vi "XYdata remove zero reduce pts.vi"(5 "reduce data pts":bool, 6 "# of final data pts":i32=5000, 7 "replace with interp. data":bool, 8 "iteration number":i32, 9 "remove zero":bool, 11 "2D input":dbl[][](array[numeric])) -> (3 "2D output":dbl[][](array[numeric]))   [LabVIEW 2020]
panel:
  # "Filter 1: Speed mode ON or OFF\nFileter 2: Remove Zero On or OFF\n    Replace with interp. data ON/OFF: When filter 2 is ON, the removed data were replaced by interpolated data"
  # "Caution: All rows will be affected."
  # "(1) Select datasets to be processed"
  # "(2) Reduce # of data if desired"
  # "(3) Select parameters for removing zeros"
  # "i) run zero-removing process?"
  # "ii) chose target column or perform for all columns"
  # "ii) after processing"
  # "delete data pts"
  # "(3) Start processing"
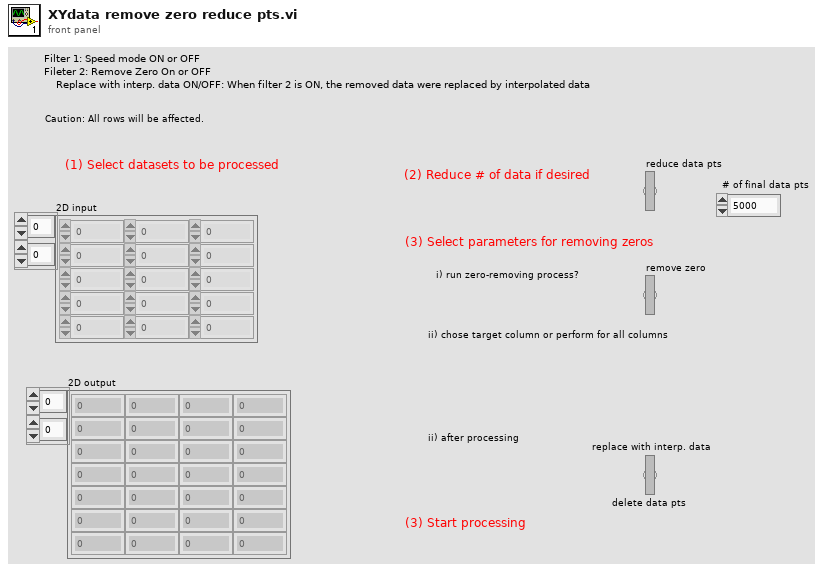
[diagram p1: front panel]
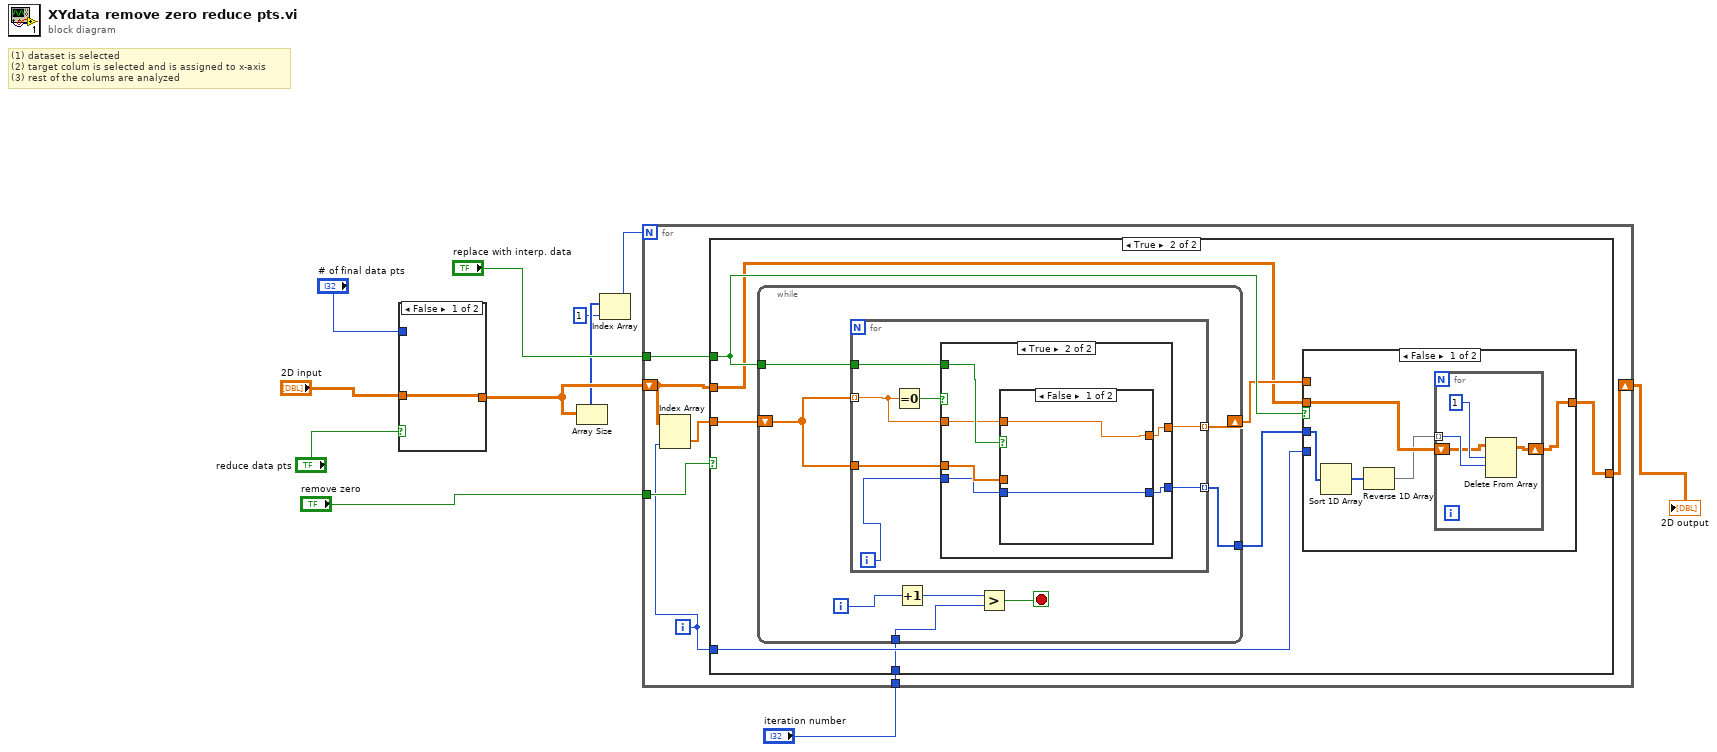
[diagram p0: block diagram]
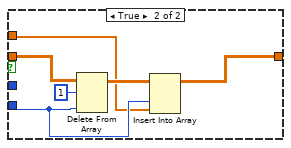
[diagram p3: hidden frame]
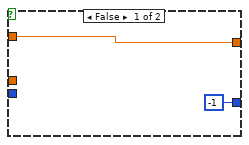
[diagram p4: hidden frame]
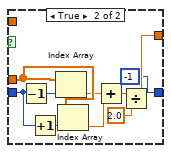
[diagram p5: hidden frame]
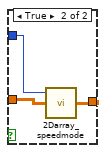
[diagram p6: hidden frame]
diagram:
  # "(1) dataset is selected\n(2) target colum is selected and is assigned to x-axis\n(3) rest of the colums are analyzed"
  n1 = case shown="False" "reduce data pts" {
    tunnel: [w12 w15] -> w8
    tunnel: "# of final data pts" -> [_ w14]
    tunnel: "2D input" -> [w12 w13]
    frame False {
    }
    frame True {
      n2 = call "2Darray_speedmode.vi"("original 2D array"=w13, "# of rows"=w14) -> ("reduced 2D array"=w15:dbl[][])  [unwired: 1 in]
    }
  }
  n3 = Array Size(array=w8) -> (size(s)=w3:i32[])
  n4 = Index Array(array=w3, index=1) -> (element=w1:i32)
  n5 = for {
    N: w1 -> [_]
    tunnel: "remove zero" -> [w22]
    tunnel: "replace with interp. data" -> [w21]
    tunnel: "iteration number" -> [w20]
    shift-right: [w19] -> w4
    shift-left: w8 -> [w16]
    i -> [w17]
    n6 = Index Array(array=w16, index (col)=w17) -> (element=w18:dbl[])  [unwired: 1 in]
    n7 = case shown="True" w22 {
      tunnel: w18 -> [_ w31]
      tunnel: [w23 w28] -> w19
      tunnel: w21 -> [_ w30]
      tunnel: w16 -> [w23 w26]
      tunnel: w17 -> [_ w25]
      tunnel: w20 -> [_ w24]
      frame False {
      }
      frame True {
        n8 = while {
          shift-right: [w53] -> w29
          shift-left: w31 -> [w54]
          tunnel: w30 -> [w49]
          tunnel: [w48] -> w27
          tunnel: w24 -> [w47]
          i -> [w52]
          stop <- w51 stop-if-true
          n9 = for {
            tunnel: w54 -> [w60] mode=indexing
            tunnel: [w61] -> w53 mode=indexing
            tunnel: w54 -> [w59]
            tunnel: w49 -> [w57]
            tunnel: [w56] -> w48 mode=indexing
            i -> [w58]
            n10 = Equal To 0?(x=w60) -> (x = 0?=w55:bool)
            n11 = case shown="True" w55 {
              tunnel: [w63 w64] -> w61
              tunnel: w60 -> [w63 w65]
              tunnel: w59 -> [_ w69]
              tunnel: w58 -> [_ w68]
              tunnel: w57 -> [_ w67]
              tunnel: [-1 w66] -> w56
              frame False {
              }
              frame True {
                n12 = case shown="False" w67 {
                  tunnel: w69 -> [_ w81]
                  tunnel: w68 -> [w71 w80]
                  tunnel: [w70 w73] -> w64
                  tunnel: [w71 -1] -> w66
                  tunnel: w65 -> [w70 _]
                  frame False {
                  }
                  frame True {
                    n13 = Decrement(x=w80) -> (x-1=w79:i32)
                    n14 = Increment(x=w80) -> (x+1=w78:i32)
                    n15 = Index Array(array=w81, index=w79) -> (element=w77:dbl)
                    n16 = Index Array(array=w81, index=w78) -> (element=w76:dbl)
                    n17 = Add(x=w77, y=w76) -> (x+y=w75:dbl)
                    n18 = Divide(x=w75, y=2.0) -> (x/y=w73:dbl)
                  }
                }
              }
            }
          }
          n19 = Increment(x=w52) -> (x+1=w50:i32)
          n20 = Greater?(x=w50, y=w47) -> (0:w51:bool)
        }
        n21 = case shown="False" w30 {
          tunnel: w29 -> [_ w42]
          tunnel: [w32 w41] -> w28
          tunnel: w26 -> [w36 w46]
          tunnel: w27 -> [w35 _]
          tunnel: w25 -> [_ w43]
          frame False {
            n22 = Sort 1D Array(array=w35) -> (sorted array=w34:i32[])
            n23 = Reverse 1D Array(array=w34) -> (reversed array=w33:i32[])
            n24 = for {
              tunnel: w33 -> [w40] mode=indexing
              shift-right: [w37] -> w32
              shift-left: w36 -> [w38]
              n25 = Delete From Array(array=w38, length=1, index (row)=w40) -> (array with subset deleted=w37:dbl[][])  [unwired: 1 in, 1 out]
            }
          }
          frame True {
            n26 = Delete From Array(array=w46, length=1, index (col)=w43) -> (array with subset deleted=w44:dbl[][])  [unwired: 1 in, 1 out]
            n27 = Insert Into Array(array=w44, index (col)=w43, new element=w42) -> (w41:dbl[][])  [unwired: 1 in]
          }
        }
      }
    }
  }
  "2D output" <- w4
